vi "sub_rplidar_inrange.vi"(8 "error in":errorcluster) -> (0 "error out":errorcluster, 3 "XY Graph":T1(graph))   [LabVIEW 2019]
uses:
  Ctrl/obstacle_info.ctl
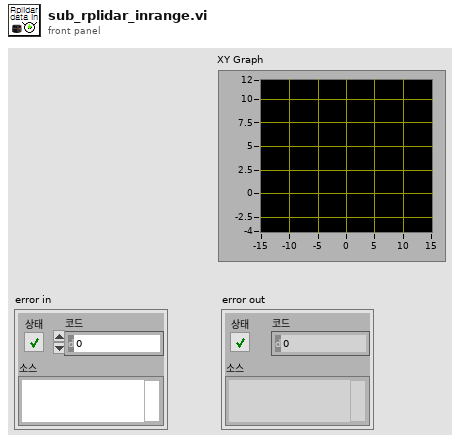
[diagram p1: front panel]
types:
  T1 = cluster{"Array out":cluster{"x":dbl, "y":dbl}[]}[]
  T2 = typedef "obstacle_info.ctl" = enum16{"init", "read", "obstacle status in", "write limit", "inrange pt-n"}
  T3 = cluster{"h range":cluster{i16, i16}, "v range":cluster{i8, i8}}
  T4 = cluster{"xy array out":cluster{"x":dbl, "y":dbl}[]}
  T5 = cluster{"limit inrange xydata":cluster{"x":dbl, "y":dbl}[]}
  T6 = cluster{"limit inrange xydata":cluster{"x":dbl, "y":dbl}[]}[]
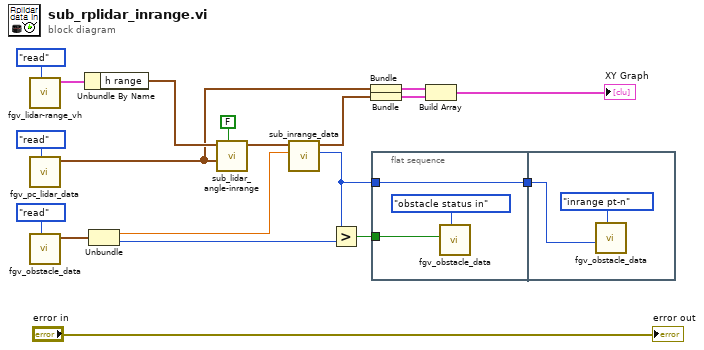
[diagram p0: block diagram]
diagram:
  n1 = call "fgv_lidar-range_vh.vi"("cmd"=enum16{"read", "write"}."read") -> ("VLP16 cfg out"=w17:T3)  [unwired: 10 in]
  n2 = call "fgv_pc_lidar_data.vi"("cmd"=enum16{"init", "read", "write"}."read") -> ("xy array out"=w3:cluster{"x":dbl, "y":dbl}[])  [unwired: 9 in, 1 out]
  n3 = call "fgv_obstacle_data.vi"("cmd"=obstacle_info."read") -> ("limit out"=w11:cluster{"RL range":dbl, "Point limit":u16})  [unwired: 7 in, 3 out]
  n4 = Unbundle By Name(w17) -> ("h range"=w7:cluster{i16, i16})
  n5 = Unbundle(w11) -> ("RL range"=w8:dbl, "Point limit"=w10:u16)
  n6 = call "sub_lidar_angle-inrange.vi"("3d"=FALSE, "2D data"=w3, "h range"=w7) -> ("Array out"=w5:cluster{"x":dbl, "y":dbl}[])  [unwired: 6 in, 2 out]
  n7 = call "sub_inrange_data.vi"("limit"=w8, "xy_lidar data"=w5) -> ("limit point out"=w14:u16, "limit inrange xydata"=w4:cluster{"x":dbl, "y":dbl}[])  [unwired: 7 in, 1 out]
  n8 = Greater?(x=w14, y=w10) -> (0:w15:bool)
  n9 = Bundle("xy array out"=w3) -> (w13:T4)  [unwired: 1 in]
  n10 = Bundle("limit inrange xydata"=w4) -> (w12:T5)  [unwired: 1 in]
  n11 = flat-sequence {
    tunnel: w15 -> [w21]
    tunnel: [w20] -> w19
    tunnel: w14 -> [w20]
    tunnel: w19 -> [w23]
    frame #0 {
      n12 = call "fgv_obstacle_data.vi"("cmd"=obstacle_info."obstacle status in", "obstacle in"=w21) -> ()  [unwired: 6 in, 4 out]
    }
    frame #1 {
      n13 = call "fgv_obstacle_data.vi"("cmd"=obstacle_info."inrange pt-n", "inrange pt-n"=w23) -> ()  [unwired: 6 in, 4 out]
    }
  }
  n14 = Build Array(w13, w12) -> (→"XY Graph":T6)
  "error out" <- "error in"
